vi "Assert Panel Main.vi"   [LabVIEW 2015, in "Login.lvclass"]
uses:
  Login.lvclass
  Member_Actor/Member_Actor/Member_Actor.lvclass
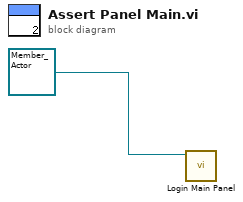
[diagram p0: block diagram]
diagram:
  n1 = call "Login Main Panel.vi"("User_Actor.lvclass"=refnum<class "Member_Actor.lvclass"> refnum ("Member_Actor.lvlib:Member_Actor.lvclass")) -> ()  [unwired: 10 in, 1 out]
